vi "NewportFlipper.vi"(9 "Settle time (ms)":dbl=1000.0, 10 "Up/Down":bool) -> ()   [LabVIEW 2022 SP3]
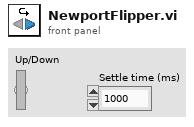
[diagram p1: front panel]
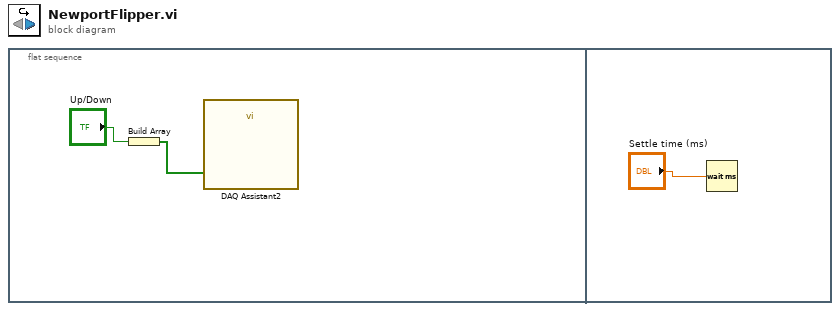
[diagram p0: block diagram]
diagram:
  n1 = flat-sequence {
    frame #0 {
      n2 = Build Array("Up/Down") -> (w1:bool[])
      n3 = call "DAQ Assistant2"("data"=w1) -> ()  [unwired: 17 in, 2 out]
    }
    frame #1 {
      n4 = Wait (ms)(milliseconds to wait="Settle time (ms)") -> ()  [unwired: 1 out]
    }
  }
